vi "Read PinMap.vi"(8 "error in (no error)":errorcluster, 11 "BML_DigiPattern_Generator in":refnum<class "DigiPattern_Generator.lvclass">) -> (0 "error out":errorcluster, 2 "PinMap":path, 3 "BML_DigiPattern_Generator out":refnum<class "DigiPattern_Generator.lvclass">)   [LabVIEW 2018, in "DigiPattern_Generator.lvclass"]
uses:
  DigiPattern_Generator.lvclass
  DigiPattern_Generator.lvclass/DigiPattern_Generator.ctl
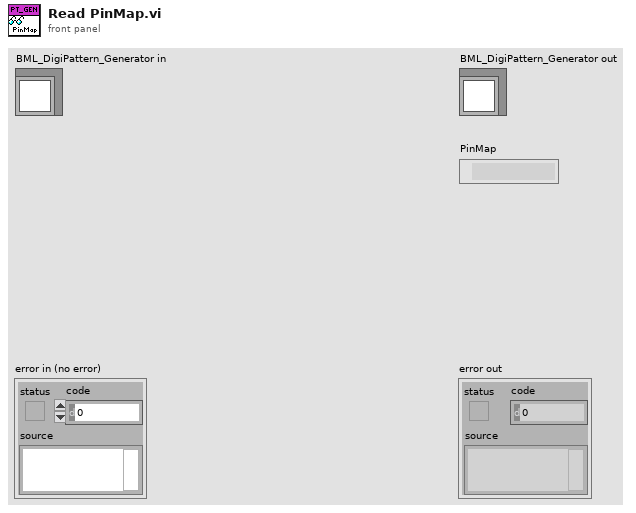
[diagram p1: front panel]
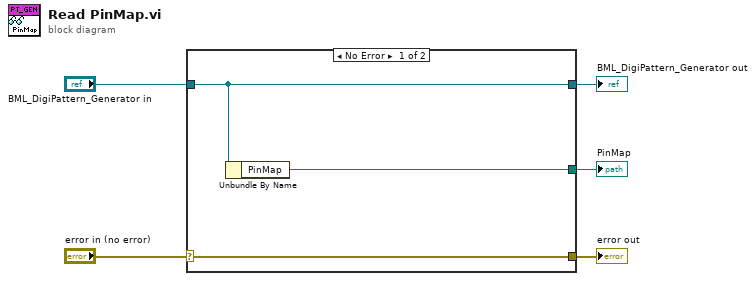
[diagram p0: block diagram]
diagram:
  n1 = case shown="No Error" "error in (no error)" {
    selector: "error in (no error)" -> [w8 w9]
    tunnel: [w8 w9] -> w4
    tunnel: [w7 w10] -> w2
    tunnel: "BML_DigiPattern_Generator in" -> [w7 w10]
    tunnel: [w6 _] -> w1
    frame No Error {
      n2 = Unbundle By Name(w7) -> ("PinMap"=w6:path)
    }
    frame Error {
    }
  }
  "error out" <- w4
  "BML_DigiPattern_Generator out" <- w2
  "PinMap" <- w1
